vi "PXI Destroy Notifiers.vi"(2 "error in (no error)":errorcluster) -> (0 "error out":errorcluster)   [LabVIEW 2015]
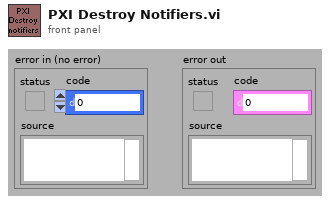
[diagram p1: front panel]
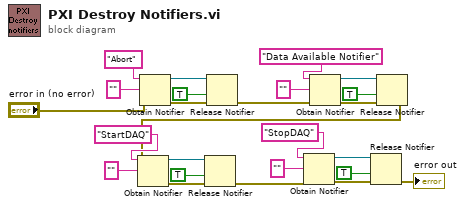
[diagram p0: block diagram]
diagram:
  n1 = Obtain Notifier(name (unnamed)="Abort", notification data type="", error in (no error)="error in (no error)") -> (notifier out=w23:refnum<notifier>, error out=w25:errorcluster)  [unwired: 1 in, 1 out]
  n2 = Release Notifier(notifier=w23, force destroy? (F)=TRUE, error in (no error)=w25) -> (error out=w14:errorcluster)  [unwired: 2 out]
  n3 = Obtain Notifier(name (unnamed)="Data Available Notifier", notification data type="", error in (no error)=w14) -> (notifier out=w19:refnum<notifier>, error out=w17:errorcluster)  [unwired: 1 in, 1 out]
  n4 = Release Notifier(notifier=w19, force destroy? (F)=TRUE, error in (no error)=w17) -> (error out=w8:errorcluster)  [unwired: 2 out]
  n5 = Obtain Notifier(name (unnamed)="StartDAQ", notification data type="", error in (no error)=w8) -> (notifier out=w11:refnum<notifier>, error out=w13:errorcluster)  [unwired: 1 in, 1 out]
  n6 = Release Notifier(notifier=w11, force destroy? (F)=TRUE, error in (no error)=w13) -> (error out=w2:errorcluster)  [unwired: 2 out]
  n7 = Obtain Notifier(name (unnamed)="StopDAQ", notification data type="", error in (no error)=w2) -> (notifier out=w5:refnum<notifier>, error out=w3:errorcluster)  [unwired: 1 in, 1 out]
  n8 = Release Notifier(notifier=w5, force destroy? (F)=TRUE, error in (no error)=w3) -> (error out=→"error out":errorcluster)  [unwired: 2 out]
